vi "RunOperation.vi"(10 "Inputs":string[](array[string]), 11 "PrintToSingleFileHtml in":refnum<class "PrintToSingleFileHtml.lvclass">) -> (1 "Output/Failure":string, 2 "CLI Process Return Code":i32, 3 "PrintToSingleFileHtml out":refnum<class "PrintToSingleFileHtml.lvclass">)   [LabVIEW 2026, in "PrintToSingleFileHtml.lvclass"]
uses:
  PrintToSingleFileHtml.lvclass
  PrintToSingleFileHtml.lvclass/PrintToSingleFileHtml.ctl
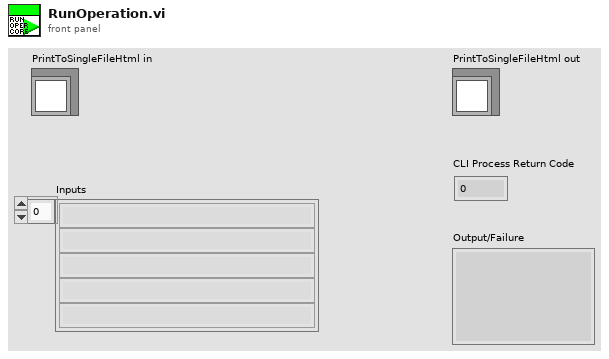
[diagram p1: front panel]
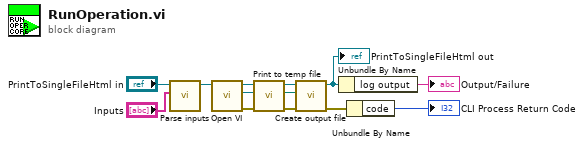
[diagram p0: block diagram]
diagram:
  n1 = call "Parse inputs.vi"("Inputs"="Inputs", "PrintToSingleFileHtml in"="PrintToSingleFileHtml in") -> ("PrintToSingleFileHtml out"=w11:refnum<class "PrintToSingleFileHtml.lvclass">)  [unwired: 9 in]
  n2 = call "Open VI.vi"("PrintToSingleFileHtml in"=w11) -> ("error out"=w7:errorcluster, "VI reference"=w8:refnum<vi>, "PrintToSingleFileHtml out"=w9:refnum<class "PrintToSingleFileHtml.lvclass">)  [unwired: 8 in]
  n3 = call "Print to temp file.vi"("error in (no error)"=w7, "VI reference"=w8, "PrintToSingleFileHtml in"=w9) -> ("error out"=w5:errorcluster, "temp file path"=w1:path, "PrintToSingleFileHtml out"=w6:refnum<class "PrintToSingleFileHtml.lvclass">)  [unwired: 6 in]
  n4 = call "Create output file.vi"("error in (no error)"=w5, "temp file path"=w1, "PrintToSingleFileHtml in"=w6) -> ("error out"=w4:errorcluster, "PrintToSingleFileHtml out"=w3:refnum<class "PrintToSingleFileHtml.lvclass">)  [unwired: 7 in]
  "PrintToSingleFileHtml out" <- w3
  n5 = Unbundle By Name(w3) -> ("log output"=→"Output/Failure":string)
  n6 = Unbundle By Name(w4) -> ("code"=→"CLI Process Return Code":i32)
